vi "On Timeout Action Camera Calibration.vi"(8 "error in (no error)":errorcluster, 11 "App in":refnum<class "App.lvclass">) -> (0 "error out":errorcluster, 3 "App out":refnum<class "App.lvclass">)   [LabVIEW 2020, in "AR Example.lvlib" / "App.lvclass"]
uses:
  App.lvclass
  App.lvclass/App.ctl
  g_ar_toolkit.capture/Stream/Stream.lvclass/Stream.ctl
  g_ar_toolkit.feature_detection/Apriltag Detector/AprilTag Detector.lvclass/AprilTag Detector.ctl
  g_ar_toolkit.image/ARGB Colour.ctl
  g_ar_toolkit.image/Draw Poly Lines (ARGB).vi
  g_ar_toolkit.image/ARGBExtractChannel.vi
  g_ar_toolkit.image/ARGB Colour to U32 Pixel Value.vi
  g_ar_toolkit.image/Draw Poly Lines (ARGB).vi/f4fe866f-059f-471d-887d-2797bd4b3b13.vi
  g_ar_toolkit.common/Module Path.vi
  <vilib>/Utility/error.llb/Error Cluster From Error Code.vi
  UI/UI.lvclass
  g_ar_toolkit.capture/Stream/Stream.lvclass
  g_ar_toolkit.image/g_ar_toolkit.image.lvlib
  g_ar_toolkit.feature_detection/Apriltag Detector/AprilTag Detector.lvclass
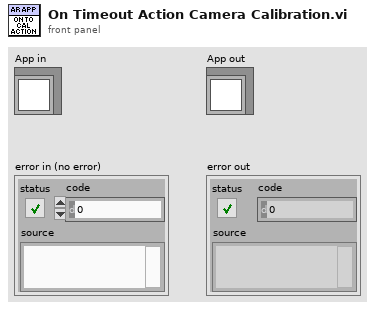
[diagram p1: front panel]
types:
  T1 = typedef "g_ar_toolkit.image.lvlib/Image Draw Offset.ctl" = cluster{"Left":i16, "Top":i16}
  T2 = typedef "g_ar_toolkit.image.lvlib/ARGB Image.ctl" = refnum<data-value>
  T3 = typedef "g_ar_toolkit.image.lvlib/ARGB Colour.ctl" = cluster{"Alpha":u8, "RGB":u32}
  T4 = typedef "g_ar_toolkit.image.lvlib/Greyscale Image.ctl" = refnum<data-value>
  T5 = typedef "g_ar_toolkit.feature_detection.lvlib/AprilTag Detector.lvclass/Detection.ctl" = cluster{"ID":i32, "Hamming":i32, "Decision Margin":sgl, "Centre":T6, "Corners":T7}
  T6 = typedef "g_ar_toolkit.common.lvlib/Image Point (Float).ctl" = cluster{"x":dbl, "y":dbl}
  T7 = typedef "g_ar_toolkit.common.lvlib/Square Corners.ctl" = cluster{"Bottom Left":T6, "Bottom Right":T6, "Top Right":T6, "Top Left":T6}
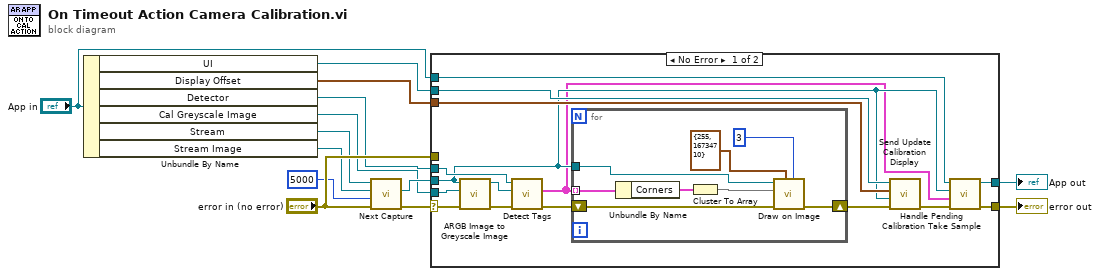
[diagram p0: block diagram]
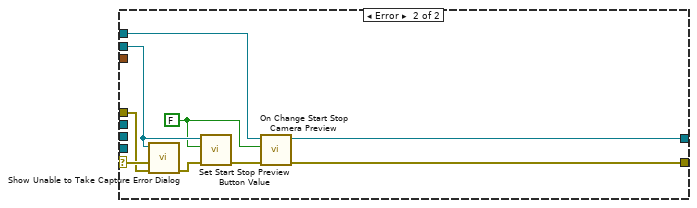
[diagram p2: hidden frame]
diagram:
  n1 = Unbundle By Name("App in") -> ("UI"=w11:refnum<class "UI.lvclass">, "Display Offset"=w8:T1, "Detector"=w1:refnum<class "AprilTag Detector.lvclass">, "Cal Greyscale Image"=w2:refnum<data-value>, "Stream"=w3:refnum<class "Stream.lvclass">, "Stream Image"=w4:refnum<data-value>)
  n2 = call "Next Capture.vi"("error in (no error)"="error in (no error)", "timeout (Default: 1000 ms)"=u16 5000 ("timeout (ms)"), "ARGB Image Destination"=w4, "Stream in"=w3) -> ("error out"=w9:errorcluster, "ARGB Image (duplicate)"=w6:T2)  [unwired: 5 in, 1 out]
  n3 = case shown="No Error" w9 {
    selector: w9 -> [w25 w42]
    tunnel: w11 -> [w28 w38]
    tunnel: [w18 w43] -> w13
    tunnel: w6 -> [w15 _]
    tunnel: "error in (no error)" -> [_ w41]
    tunnel: w8 -> [w27 _]
    tunnel: [w16 w44] -> w12
    tunnel: "App in" -> [w17 w45]
    tunnel: w2 -> [w26 _]
    tunnel: w1 -> [w24 _]
    frame No Error {
      n4 = call "ARGB Image to Greyscale Image.vi"("error in (no error)"=w25, "Greyscale Image Destination"=w26, "ARGB Image Source"=w15) -> ("error out"=w22:errorcluster, "Greyscale Image Destination (Duplicate)"=w23:T4)  [unwired: 7 in]
      n5 = call "Detect Tags.vi"("error in (no error)"=w22, "Greyscale Image"=w23, "Apriltag Detector in"=w24) -> ("error out"=w21:errorcluster, "Detections"=w14:T5[])  [unwired: 5 in, 2 out]
      n6 = for {
        tunnel: w14 -> [w33] mode=indexing
        tunnel: w15 -> [w36]
        shift-right: [w34] -> w20
        shift-left: w21 -> [w35]
        n7 = Unbundle By Name(w33) -> ("Corners"=w32:T7)
        n8 = Cluster To Array(cluster=w32) -> (array=w31:T6[])
        n9 = call-poly "Draw on Image.vi"("Thickness (Default: 1)"=3, "ARGB Colour"=T3 {"Alpha"=255, "RGB"=16734710}, "error in (no error)"=w35, "Points"=w31, "ARGB Image"=w36) -> ("error out"=w34:errorcluster)  [unwired: 5 in, 1 out]
      }
      n10 = call-dynamic "Send Update Calibration Display.vi"("error in (no error)"=w20, "Image"=w15, "Draw Offset"=w27, "UI in"=w28) -> ("error out"=w19:errorcluster)  [unwired: 7 in]
      n11 = call "Handle Pending Calibration Take Sample.vi"("error in (no error)"=w19, "Detections"=w14, "ARGB Image (duplicate)"=w15, "App in"=w17) -> ("error out"=w18:errorcluster, "App out"=w16:refnum<class "App.lvclass">)  [unwired: 6 in]
    }
    frame Error {
      w37 = FALSE ("Value")
      n12 = call-dynamic "Show Unable to Take Capture Error Dialog.vi"("error in (no error)"=w41, "Stream Start Error"=w42, "UI in"=w38) -> ("error out"=w40:errorcluster)  [unwired: 8 in]
      n13 = call-dynamic "Set Start Stop Preview Button Value.vi"("error in (no error)"=w40, "Values"=w37, "UI in"=w38) -> ("error out"=w39:errorcluster)  [unwired: 8 in]
      n14 = call "On Change Start Stop Camera Preview.vi"("error in (no error)"=w39, "Value"=w37, "App in"=w45) -> ("error out"=w43:errorcluster, "App out"=w44:refnum<class "App.lvclass">)  [unwired: 7 in]
    }
  }
  "error out" <- w13
  "App out" <- w12
